vi "Dispose.vi"(8 "error in (no error)":errorcluster, 11 "LV Awesome in":refnum<class "LV Awesome.lvclass">) -> (0 "error out":errorcluster)   [LabVIEW 2020, in "LV-Awesome.lvlib" / "LV Awesome.lvclass"]
uses:
  LV Awesome.lvclass
  LV Awesome.lvclass/LV Awesome.ctl
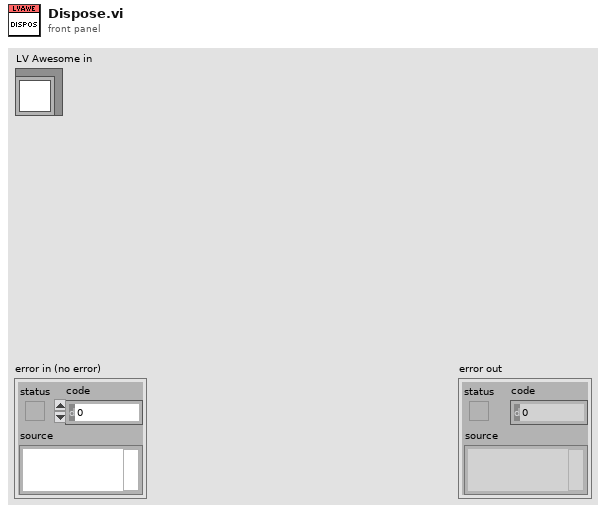
[diagram p1: front panel]
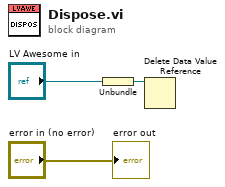
[diagram p0: block diagram]
diagram:
  n1 = Unbundle("LV Awesome in") -> (w1:refnum<data-value>)
  n2 = Delete Data Value Reference(data value reference=w1) -> ()  [unwired: 1 in, 2 out]
  "error out" <- "error in (no error)"
